vi "Create Channels.vi"(8 "error in (no error)":errorcluster, 10 "RSI Module in":refnum<class "9402.lvclass">, 11 "Parent Ref in":T1 format="%.0x") -> (0 "error out":errorcluster, 2 "RSI Module out":refnum<class "9402.lvclass">, 3 "Parent Ref out":T1 format="%.0x")   [LabVIEW 2020, in "Modules.lvlib" / "9402.lvclass"]
uses:
  9402.lvclass
  C:/Users/nitest/Desktop/Git 2020/niveristand-scan-engine-module-libraries/Source/RSI Module/RSI Module.lvclass
  <vilib>/NI VeriStand/Custom Device API/Custom Device Item Ref.ctl
  <vilib>/NI VeriStand/Custom Device API/Custom Device Channel Type.ctl
  <vilib>/NI VeriStand/Custom Device API/Custom Device Channel.ctl
  9402.lvclass/9402.ctl
  RSI Module/Class Property Strings.vi
  RSI Module/Channel GUIDs.vi
  <vilib>/NI VeriStand/Custom Device API/Custom Device API.lvlib
  RSI Module/RSI Module.lvclass
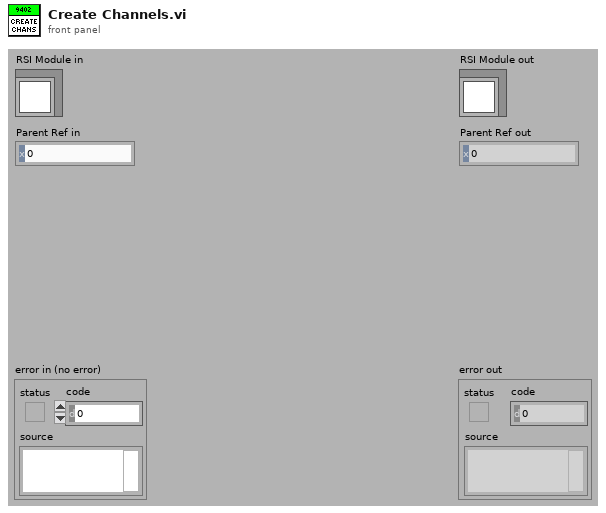
[diagram p1: front panel]
types:
  T1 = typedef "Custom Device API.lvlib/Custom Device Item Ref.ctl" = u64
  T2 = typedef "Custom Device API.lvlib/Custom Device Channel.ctl" = cluster{"Type":T3, "Units":string, "Default Value":dbl, "Faultable":bool, "Scalable":bool}
  T3 = typedef "Custom Device API.lvlib/Custom Device Channel Type.ctl" = enum16{"Input", "Output"}
  T4 = typedef "Modules.lvlib/RSI Module.lvclass/Channels.ctl" = cluster{"# Input Channels":i32, "# Output Channels":i32, "Channel Type":T5, "Units":string}
  T5 = typedef "Modules.lvlib/RSI Module.lvclass/Channel Type.ctl" = enum16{"Analog", "Digital"}
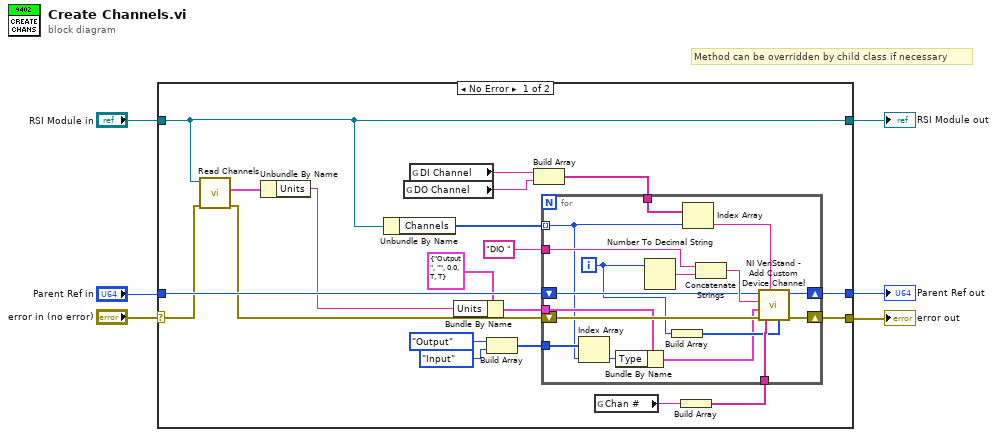
[diagram p0: block diagram]
diagram:
  # "Method can be overridden by child class if necessary"
  n1 = case shown="No Error" "error in (no error)" {
    selector: "error in (no error)" -> [w16 w46]
    tunnel: [w7 w46] -> w5
    tunnel: [w11 w45] -> w3
    tunnel: "RSI Module in" -> [w11 w45]
    tunnel: "Parent Ref in" -> [w21 w44]
    tunnel: [w8 w44] -> w1
    frame No Error {
      n2 = call "Read Channels.vi"("error in (no error)"=w16, "RSI Module in"=w11) -> ("error out"=w15:errorcluster, "Channels"=w17:T4)  [unwired: 7 in, 1 out]
      n3 = Unbundle By Name(w17) -> ("Units"=w18:string)
      n4 = Unbundle By Name(w11) -> ("Channels"=w10:u32[])
      n5 = global read "Channel GUIDs.vi" "DO Channel"() -> (w25:string)
      n6 = global read "Channel GUIDs.vi" "DI Channel"() -> (w26:string)
      n7 = Bundle By Name(cluster=T2 {"Type"=enum."Output", "Units"="", "Default Value"=0.0, "Faultable"=TRUE, "Scalable"=TRUE} ("Channel"), "Units"=w18) -> (w12:T2)
      n8 = Build Array(Custom_Device_Channel_Type."Output" ("Type"), Custom_Device_Channel_Type."Input" ("Type")) -> (w9:T3[])
      n9 = Build Array(w26, w25) -> (w22:string[])
      n10 = global read "Class Property Strings.vi" "Chan #"() -> (w20:string)
      n11 = Build Array(w20) -> (w19:string[])
      n12 = for {
        tunnel: "DIO " ("Channel Name") -> [w41]
        tunnel: w12 -> [w32]
        tunnel: w22 -> [w34]
        tunnel: w19 -> [w38]
        shift-right: [w36] -> w7
        shift-left: w15 -> [w42]
        shift-right: [w35] -> w8
        shift-left: w21 -> [w39]
        tunnel: w10 -> [w27] mode=indexing
        tunnel: w9 -> [w31]
        i -> [w28]
        n13 = Index Array(array=w31, index=w27) -> (element=w30:T3)
        n14 = Bundle By Name(cluster=w32, "Type"=w30) -> (w29:T2)
        n15 = Number To Decimal String(number=w28) -> (decimal integer string=w43:string)  [unwired: 1 in]
        n16 = Build Array(w28) -> (w37:i32[])
        n17 = Index Array(array=w34, index=w27) -> (element=w33:string)
        n18 = Concatenate Strings(w41, w43) -> (w40:string)
        n19 = call <vilib>:"NI VeriStand - Add Custom Device Channel.vi"("Property Values"=w37, "Property names"=w38, "GUID (Default Channel)"=w33, "error in (no error)"=w42, "Channel"=w29, "Channel Name"=w40, "Parent Ref in"=w39) -> ("error out"=w36:errorcluster, "Parent Ref out"=w35:T1)  [unwired: 1 in, 2 out]
      }
    }
    frame Error {
    }
  }
  "error out" <- w5
  "RSI Module out" <- w3
  "Parent Ref out" <- w1
